vi "Write Output Directory.vi"(8 "error in (no error)":errorcluster, 10 "Output Directory":path, 11 "SG Path in":refnum<class "SG 18GHz Path.lvclass">) -> (0 "error out":errorcluster, 3 "SG Path out":refnum<class "SG 18GHz Path.lvclass">)   [LabVIEW 2023, in "RFFixtureCharact.RFPM.lvlib" / "SG 18GHz Path.lvclass"]
uses:
  SG 18GHz Path.lvclass
  SG 18GHz Path.lvclass/SG 18GHz Path.ctl
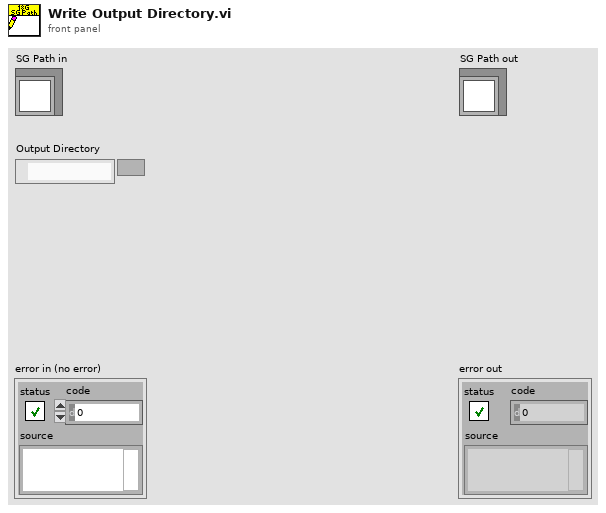
[diagram p1: front panel]
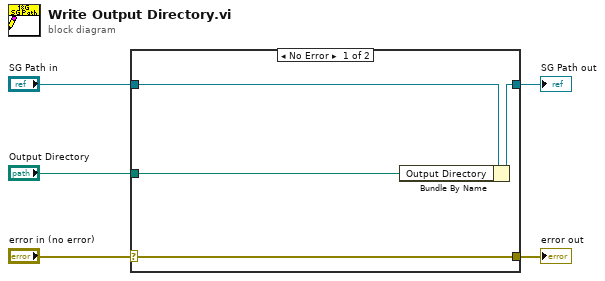
[diagram p0: block diagram]
diagram:
  n1 = case shown="No Error" "error in (no error)" {
    selector: "error in (no error)" -> [w9 w10]
    tunnel: [w9 w10] -> w4
    tunnel: [w7 w11] -> w2
    tunnel: "SG Path in" -> [w8 w11]
    tunnel: "Output Directory" -> [w6 _]
    frame No Error {
      n2 = Bundle By Name(cluster=w8, "Output Directory"=w6) -> (w7:refnum<class "SG 18GHz Path.lvclass">)
    }
    frame Error {
    }
  }
  "error out" <- w4
  "SG Path out" <- w2
